vi "KlingerV2 SetAxisParams.vi"(0 "Axe":u8(ring) items=["W", "X", "Y", "Z"], 1 "TypeMouv":i32(ring) caption="Type de mouvement" items=["Linéaire", "Rotation"], 2 "Nom de l'axe":string, 3 "Speed":cluster{"Vitesse":i32, "Accel":dbl}={"Vitesse"=800, "Accel"=0.4000000059604645} {"Accel" min=0.10000000149011612 max=2.0 step=0.10000000149011612 format="%#.1f"; "Vitesse" min=32 max=4000 step=1 format="%#.0f"}, 4 "Param":T1, 5 "Type":i32(ring) caption="Type de moteur" items=["UE30", "UE72"], 7 "FactConv":dbl=0.01 caption="Facteur de\nConversion\n(m/pas ou °/pas)" format="%#_7g", 9 "CorrParams":T2={"CorrActive"=FALSE, "ErreurLim"=0.1, "NbrEssais"=3} caption="Paramètres de correction de position" {"NbrEssais" min=1 max=5 step=1; "ErreurLim" min=0.0 max=10.0 step=0.1 format="%#.1f"}, 11 "error in":errorcluster, 12 "Encodeur":bool caption="Possède un\nEncodeur", 13 "Origine":bool caption="Possède un\nInterrupteur d'origine", 14 "Id Num":i32 caption="Numéro Id.") -> (15 "error out":errorcluster)   [LabVIEW 2012]
doc: "Ce Vi enregistre les paramètres des différents axes dans un fichier .ini"
uses:
  <userlib>/KlingerV2/KlingerV2 Params.ctl
  <vilib>/Utility/config.llb/Write Key (I32).vi
  <vilib>/Utility/config.llb/Write Key (Double).vi
  <vilib>/Utility/config.llb/Write Key (Boolean).vi
  <vilib>/Utility/config.llb/Read Key (I32).vi
  <vilib>/Utility/config.llb/Write Key (String).vi
  <vilib>/Utility/config.llb/NI_LVConfig.lvlib
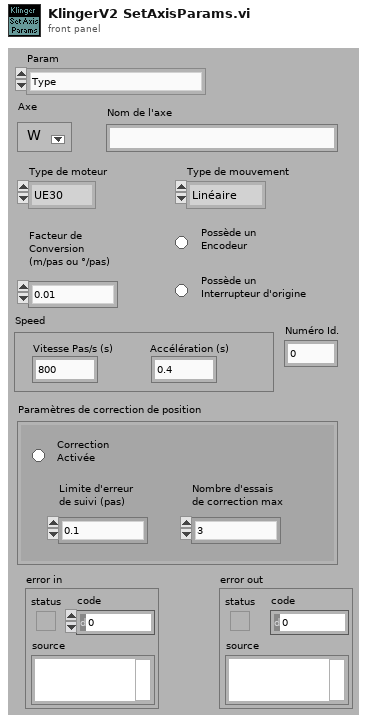
[diagram p1: front panel]
types:
  T1 = typedef "KlingerV2 Params.ctl" = enum16{"Type", "Origine", "Encodeur", "TypeMouv", "FactConv", "Nom", "CorrParams", "KlingCtrlPar", "Speed", "Acc", "Avance", "Tous"}
  T2 = cluster{"CorrActive":bool, "ErreurLim":dbl, "NbrEssais":i32}
  T3 = typedef "NI_LVConfig.lvlib/Config Data RefNum.ctl" = refnum<k1>
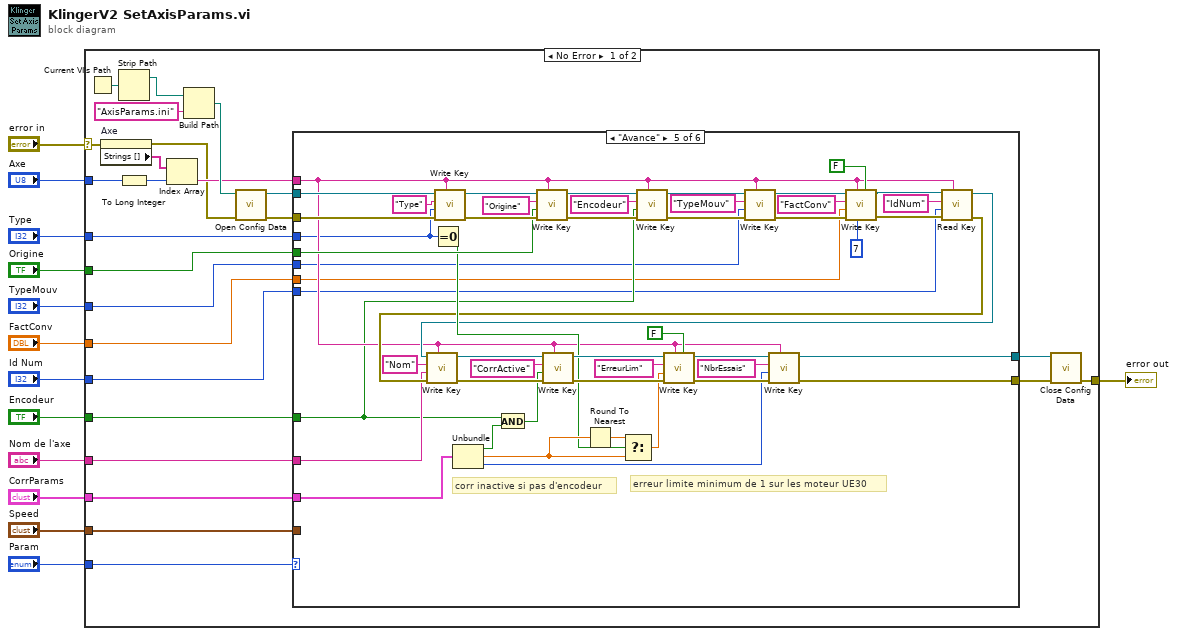
[diagram p0: block diagram]
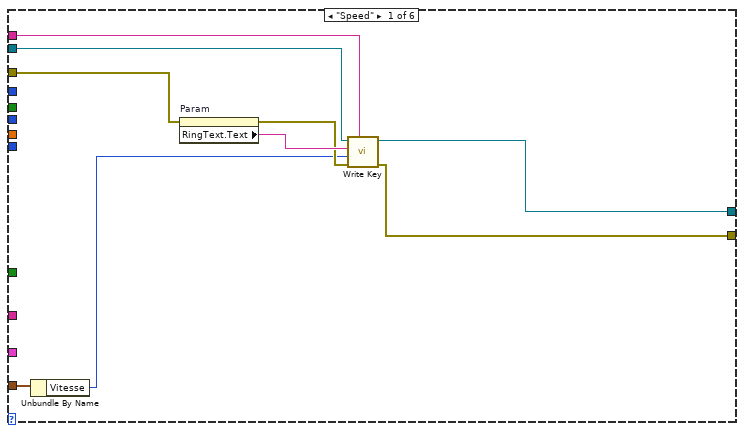
[diagram p2: hidden frame]
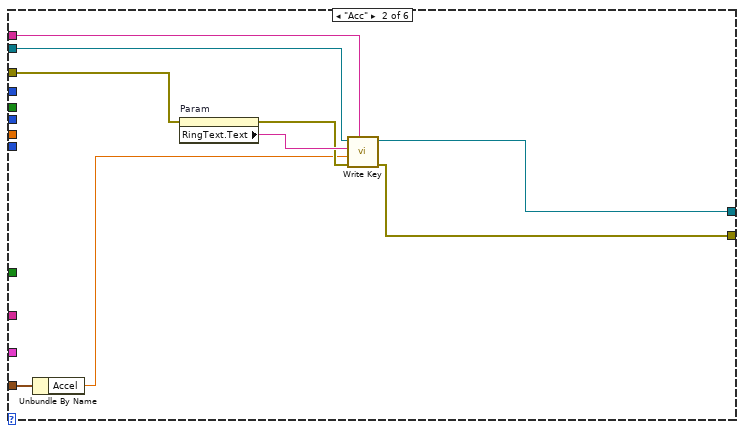
[diagram p3: hidden frame]
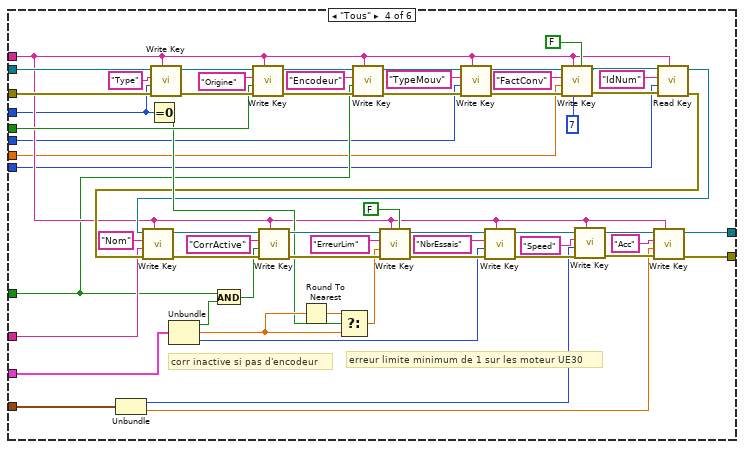
[diagram p5: hidden frame]
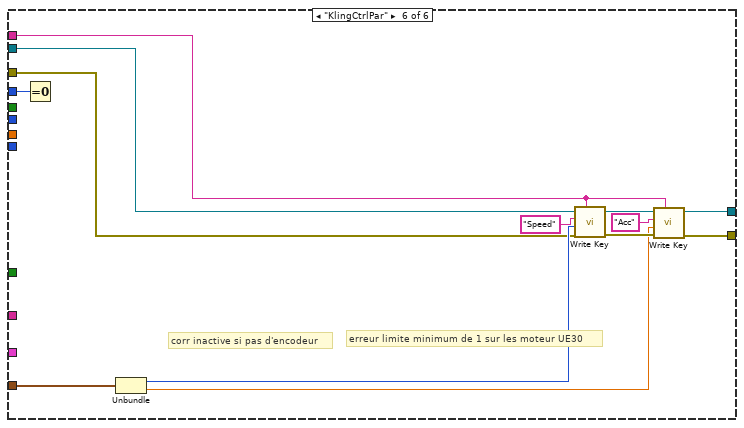
[diagram p6: hidden frame]
diagram:
  n1 = case shown="No Error" "error in" {
    selector: "error in" -> [w23 w183]
    tunnel: "Axe" -> [w35 _]
    tunnel: [w30 w183] -> w12
    tunnel: "Param" -> [w26 _]
    tunnel: "Origine" -> [w25 _]
    tunnel: "Type" -> [w21 _]
    tunnel: "Speed" -> [w20 _]
    tunnel: "CorrParams" -> [w19 _]
    tunnel: "Nom de l'axe" -> [w18 _]
    tunnel: "Encodeur" -> [w17 _]
    tunnel: "TypeMouv" -> [w16 _]
    tunnel: "FactConv" -> [w15 _]
    tunnel: "Id Num" -> [w14 _]
    frame No Error {
      n2 = Current VI's Path() -> (path=w38:path)
      n3 = property on="Axe" class="Ring (strict)"(error in=w23) -> (error out=w22:errorcluster, "Strings []"=w33:string[])  [unwired: 1 in, 1 out]
      n4 = Strip Path(path=w38) -> (stripped path=w24:path)  [unwired: 1 out]
      n5 = To Long Integer(number=w35) -> (32bit integer=w34:i32)
      n6 = Index Array(array=w33, index=w34) -> (element=w29:string)
      n7 = Build Path(base path=w24, name or relative path="AxisParams.ini") -> (appended path=w36:path)
      n8 = call <vilib>:"Open Config Data.vi"("error in (no error)"=w22, "configuration file path"=w36) -> ("error out"=w31:errorcluster, "refnum"=w32:T3)  [unwired: 7 in, 1 out]
      n9 = case shown="\"Avance\"" w26 {
        tunnel: w32 -> [w39 w48 w58 w110 w161 w172]
        tunnel: w31 -> [w44 w53 w57 w109 w160 w171]
        tunnel: w25 -> [_ _ _ w99 w150 _]
        tunnel: w29 -> [w47 w56 _ w67 w128 w170]
        tunnel: [w43 w52 w57 w70 w119 w177] -> w28
        tunnel: [w42 w51 w58 w69 w120 w176] -> w27
        tunnel: w21 -> [_ _ _ w66 w127 w174]
        tunnel: w20 -> [w41 w50 _ w65 _ w173]
        tunnel: w19 -> [_ _ _ w64 w126 _]
        tunnel: w18 -> [_ _ _ w63 w125 _]
        tunnel: w17 -> [_ _ _ w62 w124 _]
        tunnel: w16 -> [_ _ _ w61 w123 _]
        tunnel: w15 -> [_ _ _ w60 w122 _]
        tunnel: w14 -> [_ _ _ w59 w121 _]
        frame "Speed" {
          n10 = Unbundle By Name(w41) -> ("Vitesse"=w40:i32)
          n11 = property on="Param" class="Enum (strict)"(error in=w44) -> (error out=w45:errorcluster, "RingText.Text"=w46:string)  [unwired: 1 in, 1 out]
          n12 = call-poly <vilib>:"Write Key.vi"("section"=w47, "error in (no error)"=w45, "value"=w40, "key"=w46, "refnum"=w39) -> ("error out"=w43:errorcluster, "refnum out"=w42:T3)  [unwired: 4 in, 1 out]
        }
        frame "Acc" {
          n13 = Unbundle By Name(w50) -> ("Accel"=w49:dbl)
          n14 = property on="Param" class="Enum (strict)"(error in=w53) -> (error out=w54:errorcluster, "RingText.Text"=w55:string)  [unwired: 1 in, 1 out]
          n15 = call-poly <vilib>:"Write Key.vi"("section"=w56, "error in (no error)"=w54, "value"=w49, "key"=w55, "refnum"=w48) -> ("error out"=w52:errorcluster, "refnum out"=w51:T3)  [unwired: 4 in, 1 out]
        }
        frame Default {
          # "choix invalide!"
        }
        frame "Tous" {
          # "erreur limite minimum de 1 sur les moteur UE30"
          # "corr inactive si pas d'encodeur"
          n16 = Unbundle(w65) -> ("Vitesse"=w80:i32, "Accel"=w68:dbl)
          n17 = Equal To 0?(x=w66) -> (x = 0?=w88:bool)
          n18 = call-poly <vilib>:"Write Key.vi"("section"=w67, "error in (no error)"=w109, "value"=w66, "key"="Type", "refnum"=w110) -> ("error out"=w106:errorcluster, "refnum out"=w108:T3)  [unwired: 4 in, 1 out]
          n19 = Unbundle(w64) -> ("CorrActive"=w87:bool, "ErreurLim"=w90:dbl, "NbrEssais"=w92:i32)
          n20 = And(x=w62, y=w87) -> (x .and. y?=w86:bool)
          n21 = call-poly <vilib>:"Write Key.vi"("section"=w67, "error in (no error)"=w106, "value"=w99, "key"="Origine", "refnum"=w108) -> ("error out"=w105:errorcluster, "refnum out"=w100:T3)  [unwired: 4 in, 1 out]
          n22 = Round To Nearest(number=w90) -> (nearest integer value=w91:dbl)
          n23 = Select(t=w91, s=w88, f=w90) -> (s? t:f=w89:dbl)
          n24 = call-poly <vilib>:"Write Key.vi"("section"=w67, "error in (no error)"=w105, "value"=w62, "key"="Encodeur", "refnum"=w100) -> ("error out"=w104:errorcluster, "refnum out"=w101:T3)  [unwired: 4 in, 1 out]
          n25 = call-poly <vilib>:"Write Key.vi"("section"=w67, "error in (no error)"=w104, "value"=w61, "key"="TypeMouv", "refnum"=w101) -> ("error out"=w103:errorcluster, "refnum out"=w102:T3)  [unwired: 4 in, 1 out]
          n26 = call-poly <vilib>:"Write Key.vi"("use system decimal point (T)"=FALSE, "precision (6)"=i16 7, "section"=w67, "error in (no error)"=w103, "value"=w60, "key"="FactConv", "refnum"=w102) -> ("error out"=w75:errorcluster, "refnum out"=w74:T3)  [unwired: 2 in, 1 out]
          n27 = call-poly <vilib>:"Read Key.vi"("section"=w67, "error in (no error)"=w75, "default value"=w59, "key"="IdNum", "refnum"=w74) -> ("error out"=w77:errorcluster, "refnum out"=w76:T3)  [unwired: 3 in, 2 out]
          n28 = call-poly <vilib>:"Write Key.vi"("section"=w67, "error in (no error)"=w77, "value"=w63, "key"="Nom", "refnum"=w76) -> ("error out"=w97:errorcluster, "refnum out"=w98:T3)  [unwired: 4 in, 1 out]
          n29 = call-poly <vilib>:"Write Key.vi"("section"=w67, "error in (no error)"=w97, "value"=w86, "key"="CorrActive", "refnum"=w98) -> ("error out"=w95:errorcluster, "refnum out"=w96:T3)  [unwired: 4 in, 1 out]
          n30 = call-poly <vilib>:"Write Key.vi"("use system decimal point (T)"=FALSE, "section"=w67, "error in (no error)"=w95, "value"=w89, "key"="ErreurLim", "refnum"=w96) -> ("error out"=w93:errorcluster, "refnum out"=w94:T3)  [unwired: 3 in, 1 out]
          n31 = call-poly <vilib>:"Write Key.vi"("section"=w67, "error in (no error)"=w93, "value"=w92, "key"="NbrEssais", "refnum"=w94) -> ("error out"=w82:errorcluster, "refnum out"=w81:T3)  [unwired: 4 in, 1 out]
          n32 = call-poly <vilib>:"Write Key.vi"("section"=w67, "error in (no error)"=w82, "value"=w80, "key"="Speed", "refnum"=w81) -> ("error out"=w71:errorcluster, "refnum out"=w72:T3)  [unwired: 4 in, 1 out]
          n33 = call-poly <vilib>:"Write Key.vi"("section"=w67, "error in (no error)"=w71, "value"=w68, "key"="Acc", "refnum"=w72) -> ("error out"=w70:errorcluster, "refnum out"=w69:T3)  [unwired: 4 in, 1 out]
        }
        frame "Avance" {
          # "erreur limite minimum de 1 sur les moteur UE30"
          # "corr inactive si pas d'encodeur"
          n34 = Equal To 0?(x=w127) -> (x = 0?=w139:bool)
          n35 = call-poly <vilib>:"Write Key.vi"("section"=w128, "error in (no error)"=w160, "value"=w127, "key"="Type", "refnum"=w161) -> ("error out"=w157:errorcluster, "refnum out"=w159:T3)  [unwired: 4 in, 1 out]
          n36 = Unbundle(w126) -> ("CorrActive"=w138:bool, "ErreurLim"=w141:dbl, "NbrEssais"=w143:i32)
          n37 = And(x=w124, y=w138) -> (x .and. y?=w137:bool)
          n38 = call-poly <vilib>:"Write Key.vi"("section"=w128, "error in (no error)"=w157, "value"=w150, "key"="Origine", "refnum"=w159) -> ("error out"=w156:errorcluster, "refnum out"=w151:T3)  [unwired: 4 in, 1 out]
          n39 = Round To Nearest(number=w141) -> (nearest integer value=w142:dbl)
          n40 = Select(t=w142, s=w139, f=w141) -> (s? t:f=w140:dbl)
          n41 = call-poly <vilib>:"Write Key.vi"("section"=w128, "error in (no error)"=w156, "value"=w124, "key"="Encodeur", "refnum"=w151) -> ("error out"=w155:errorcluster, "refnum out"=w152:T3)  [unwired: 4 in, 1 out]
          n42 = call-poly <vilib>:"Write Key.vi"("section"=w128, "error in (no error)"=w155, "value"=w123, "key"="TypeMouv", "refnum"=w152) -> ("error out"=w154:errorcluster, "refnum out"=w153:T3)  [unwired: 4 in, 1 out]
          n43 = call-poly <vilib>:"Write Key.vi"("use system decimal point (T)"=FALSE, "precision (6)"=i16 7, "section"=w128, "error in (no error)"=w154, "value"=w122, "key"="FactConv", "refnum"=w153) -> ("error out"=w130:errorcluster, "refnum out"=w129:T3)  [unwired: 2 in, 1 out]
          n44 = call-poly <vilib>:"Read Key.vi"("section"=w128, "error in (no error)"=w130, "default value"=w121, "key"="IdNum", "refnum"=w129) -> ("error out"=w132:errorcluster, "refnum out"=w131:T3)  [unwired: 3 in, 2 out]
          n45 = call-poly <vilib>:"Write Key.vi"("section"=w128, "error in (no error)"=w132, "value"=w125, "key"="Nom", "refnum"=w131) -> ("error out"=w148:errorcluster, "refnum out"=w149:T3)  [unwired: 4 in, 1 out]
          n46 = call-poly <vilib>:"Write Key.vi"("section"=w128, "error in (no error)"=w148, "value"=w137, "key"="CorrActive", "refnum"=w149) -> ("error out"=w146:errorcluster, "refnum out"=w147:T3)  [unwired: 4 in, 1 out]
          n47 = call-poly <vilib>:"Write Key.vi"("use system decimal point (T)"=FALSE, "section"=w128, "error in (no error)"=w146, "value"=w140, "key"="ErreurLim", "refnum"=w147) -> ("error out"=w144:errorcluster, "refnum out"=w145:T3)  [unwired: 3 in, 1 out]
          n48 = call-poly <vilib>:"Write Key.vi"("section"=w128, "error in (no error)"=w144, "value"=w143, "key"="NbrEssais", "refnum"=w145) -> ("error out"=w119:errorcluster, "refnum out"=w120:T3)  [unwired: 4 in, 1 out]
        }
        frame "KlingCtrlPar" {
          # "erreur limite minimum de 1 sur les moteur UE30"
          # "corr inactive si pas d'encodeur"
          n49 = Equal To 0?(x=w174) -> ()  [unwired: 1 out]
          n50 = Unbundle(w173) -> ("Vitesse"=w182:i32, "Accel"=w175:dbl)
          n51 = call-poly <vilib>:"Write Key.vi"("section"=w170, "error in (no error)"=w171, "value"=w182, "key"="Speed", "refnum"=w172) -> ("error out"=w178:errorcluster, "refnum out"=w179:T3)  [unwired: 4 in, 1 out]
          n52 = call-poly <vilib>:"Write Key.vi"("section"=w170, "error in (no error)"=w178, "value"=w175, "key"="Acc", "refnum"=w179) -> ("error out"=w177:errorcluster, "refnum out"=w176:T3)  [unwired: 4 in, 1 out]
        }
      }
      n53 = call <vilib>:"Close Config Data.vi"("error in (no error)"=w28, "refnum"=w27) -> ("error out"=w30:errorcluster)  [unwired: 8 in, 1 out]
    }
    frame Error {
    }
  }
  "error out" <- w12
